vi "Input convert (SubVI).vi"(11 "Signals in":dbl[](array[numeric])) -> (2 "Nu mes":dbl[](array[numeric]), 3 "Eta mes":dbl[](array[numeric]), 5 "heading":dbl)   [LabVIEW 2014]
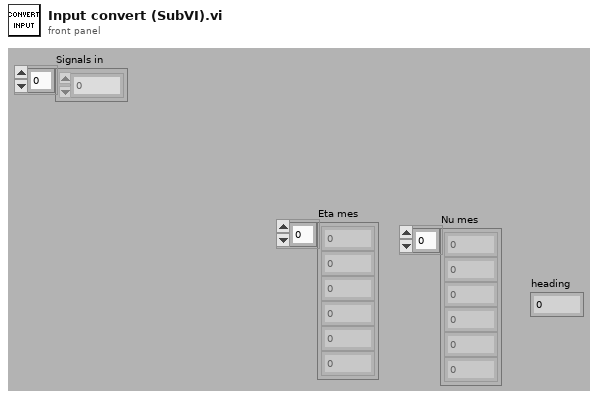
[diagram p1: front panel]
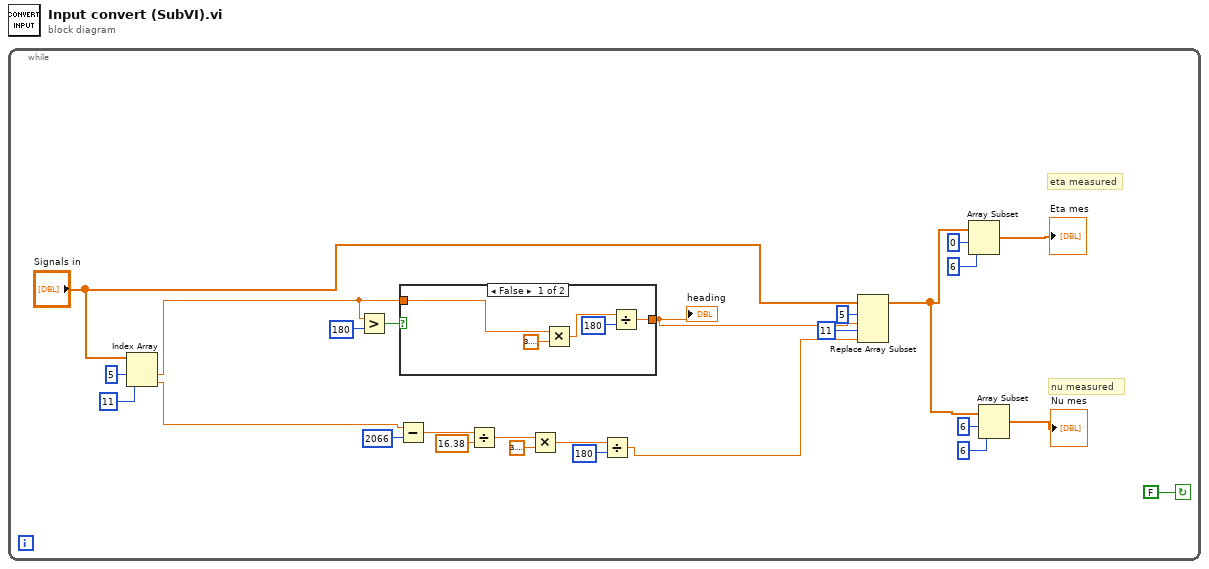
[diagram p0: block diagram]
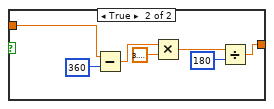
[diagram p2: hidden frame]
diagram:
  n1 = while {
    stop <- FALSE continue-if-true
    # "eta measured"
    # "nu measured"
    n2 = Index Array(array="Signals in", index #1=5 ("index"), index #2=11 ("index")) -> (element #1=w15:dbl, element #2=w13:dbl)
    n3 = Greater?(x=w15, y=180) -> (0:w25:bool)
    n4 = Subtract(x=w13, y=2066) -> (x-y=w18:dbl)
    n5 = case shown="False" w25 {
      tunnel: [w28 w33] -> w10
      tunnel: w15 -> [w27 w32]
      frame False {
        n6 = Multiply(x=w27, y=3.141592653589793) -> (x*y=w29:dbl)
        n7 = Divide(x=w29, y=180) -> (x/y=w28:dbl)
      }
      frame True {
        n8 = Subtract(x=w32, y=360) -> (x-y=w34:dbl)
        n9 = Multiply(x=w34, y=3.141592653589793) -> (x*y=w38:dbl)
        n10 = Divide(x=w38, y=180) -> (x/y=w33:dbl)
      }
    }
    "heading" <- w10
    n11 = Divide(x=w18, y=16.38) -> (x/y=w21:dbl)
    n12 = Multiply(x=w21, y=3.141592653589793) -> (x*y=w23:dbl)
    n13 = Divide(x=w23, y=180) -> (x/y=w8:dbl)
    n14 = Replace Array Subset(array="Signals in", new element #1=w10, index #1=5 ("index"), new element #2=w8, index #2=11 ("index")) -> (w3:dbl[])
    n15 = Array Subset(array=w3, index=0, length=6) -> (→"Eta mes":dbl[])
    n16 = Array Subset(array=w3, index=6, length=6) -> (→"Nu mes":dbl[])
  }
